vi "goToNextValue.vi"(5 "maxValue":i32, 7 "min Value":i32, 9 "value in":i32, 11 "Values Pool":i32[](array[numeric])) -> (1 "next value":i32, 3 "RolledOver":bool)   [LabVIEW 2013, in "openCron.lvlib" / "Cron.lvclass"]
uses:
  Cron.lvclass
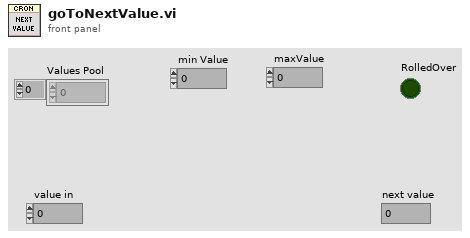
[diagram p1: front panel]
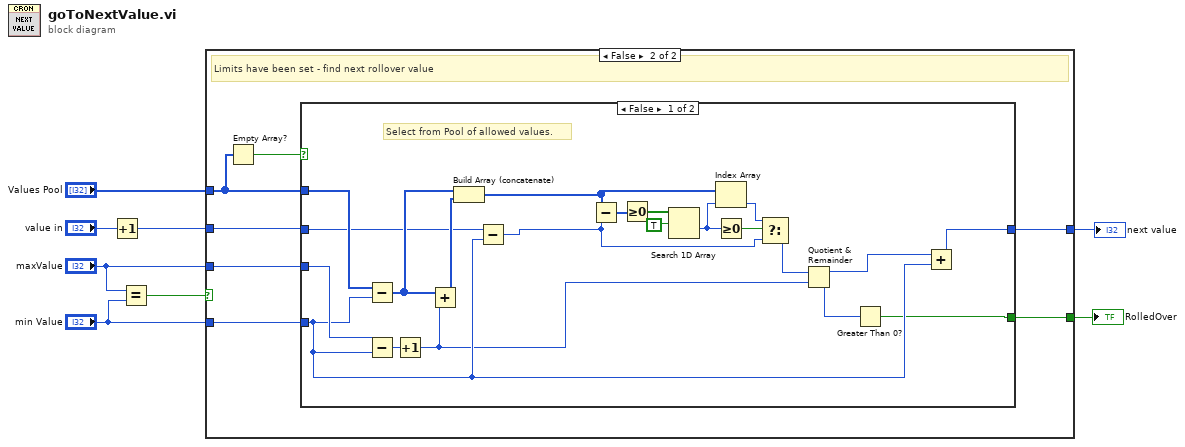
[diagram p0: block diagram]
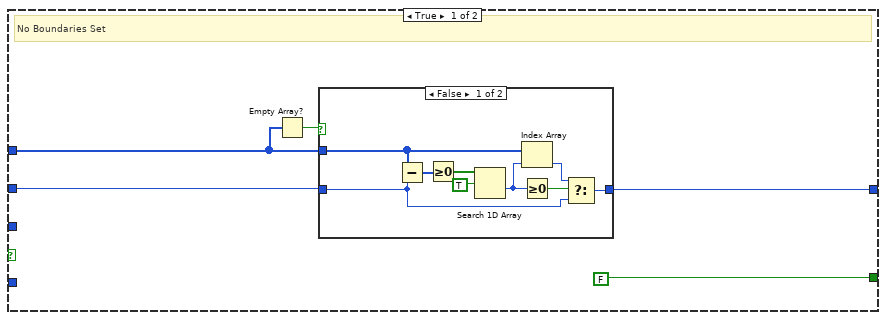
[diagram p2: hidden frame]
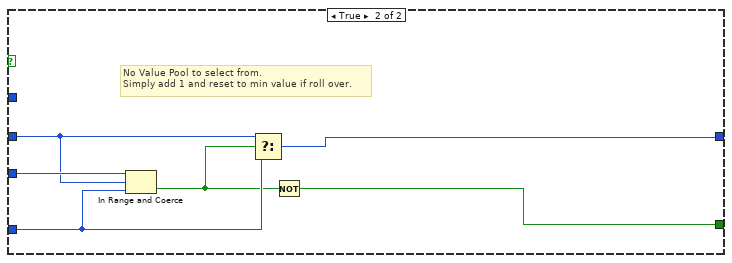
[diagram p4: hidden frame]
diagram:
  n1 = Increment(x="value in") -> (x+1=w6:i32)
  n2 = Equal?(x="maxValue", y="min Value") -> (x = y?=w4:bool)
  n3 = case shown="False" w4 {
    tunnel: "Values Pool" -> [w13 w29]
    tunnel: w6 -> [w11 w28]
    tunnel: [w10 w24] -> w5
    tunnel: "maxValue" -> [_ w27]
    tunnel: "min Value" -> [_ w26]
    tunnel: [FALSE w25] -> w1
    frame True {
      # "No Boundaries Set"
      n4 = Empty Array?(array=w13) -> (empty?=w12:bool)
      n5 = case shown="False" w12 {
        tunnel: w11 -> [w15 w23]
        tunnel: [w18 w23] -> w10
        tunnel: w13 -> [w19 _]
        frame False {
          n6 = Subtract(x=w19, y=w15) -> (x-y=w22:i32[])
          n7 = Greater Or Equal To 0?(x=w22) -> (x >= 0?=w21:bool[])
          n8 = Search 1D Array(1D array=w21, element=TRUE) -> (index of element=w14:i32)  [unwired: 1 in]
          n9 = Index Array(array=w19, index=w14) -> (element=w16:i32)
          n10 = Greater Or Equal To 0?(x=w14) -> (x >= 0?=w17:bool)
          n11 = Select(t=w16, s=w17, f=w15) -> (s? t:f=w18:i32)
        }
        frame True {
        }
      }
    }
    frame False {
      # "Limits have been set - find next rollover value"
      n12 = Empty Array?(array=w29) -> (empty?=w30:bool)
      n13 = case shown="False" w30 {
        tunnel: w28 -> [w39 w56]
        tunnel: [w36 w54] -> w24
        tunnel: w29 -> [w42 _]
        tunnel: w27 -> [w44 w57]
        tunnel: w26 -> [w37 w55]
        tunnel: [w31 w52] -> w25
        frame False {
          # "Select from Pool of allowed values."
          n14 = Subtract(x=w42, y=w37) -> (x-y=w41:i32[])
          n15 = Subtract(x=w44, y=w37) -> (x-y=w43:i32)
          n16 = Increment(x=w43) -> (x+1=w35:i32)
          n17 = Add(x=w41, y=w35) -> (x+y=w40:i32[])
          n18 = Build Array (concatenate)(w41, w40) -> (w45:i32[])
          n19 = Subtract(x=w39, y=w37) -> (x-y=w38:i32)
          n20 = Subtract(x=w45, y=w38) -> (x-y=w51:i32[])
          n21 = Greater Or Equal To 0?(x=w51) -> (x >= 0?=w50:bool[])
          n22 = Search 1D Array(1D array=w50, element=TRUE) -> (index of element=w46:i32)  [unwired: 1 in]
          n23 = Index Array(array=w45, index=w46) -> (element=w47:i32)
          n24 = Greater Or Equal To 0?(x=w46) -> (x >= 0?=w48:bool)
          n25 = Select(t=w47, s=w48, f=w38) -> (s? t:f=w34:i32)
          n26 = Quotient & Remainder(x=w34, y=w35) -> (x-y*floor(x/y)=w33:i32, floor(x/y)=w32:i32)
          n27 = Greater Than 0?(x=w32) -> (x > 0?=w31:bool)
          n28 = Add(x=w33, y=w37) -> (x+y=w36:i32)
        }
        frame True {
          # "No Value Pool to select from.\nSimply add 1 and reset to min value if roll over."
          n29 = In Range and Coerce(upper limit=w57, x=w56, lower limit=w55) -> (In Range?=w53:bool)  [unwired: 1 out]
          n30 = Select(t=w56, s=w53, f=w55) -> (s? t:f=w54:i32)
          n31 = Not(x=w53) -> (.not. x?=w52:bool)
        }
      }
    }
  }
  "next value" <- w5
  "RolledOver" <- w1
